vi "Set Home State.vi"(8 "error in (no error)":errorcluster, 9 "Home?":bool, 10 "Motor":i32, 11 "Filter Wheel in":refnum<class "Filter Wheel.lvclass">) -> (0 "error out":errorcluster, 3 "Filter Wheel out":refnum<class "Filter Wheel.lvclass">)   [LabVIEW 2024, in "Filter Wheel.lvclass"]
uses:
  Filter Wheel.lvclass
  Filter Wheel.lvclass/Filter Wheel.ctl
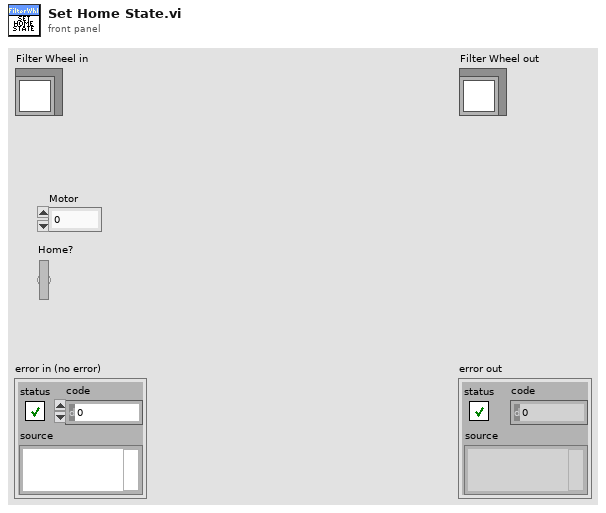
[diagram p1: front panel]
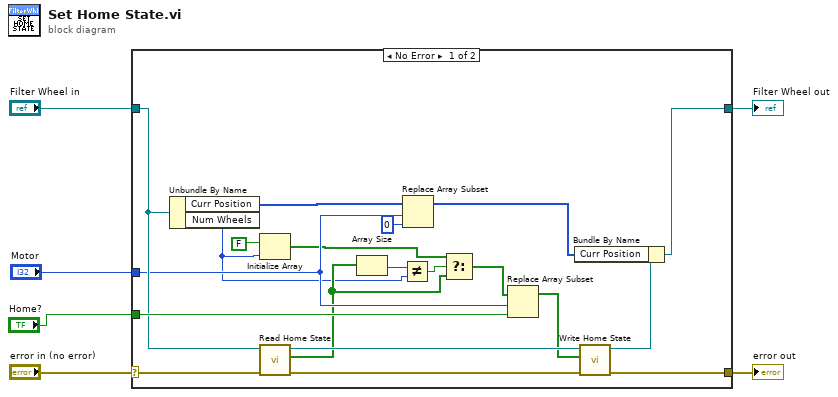
[diagram p0: block diagram]
diagram:
  n1 = case shown="No Error" "error in (no error)" {
    selector: "error in (no error)" -> [w24 w28]
    tunnel: [w22 w28] -> w5
    tunnel: [w19 w27] -> w3
    tunnel: "Filter Wheel in" -> [w18 w27]
    tunnel: "Motor" -> [w16 _]
    tunnel: "Home?" -> [w21 _]
    frame No Error {
      n2 = Unbundle By Name(w18) -> ("Curr Position"=w17:i32[], "Num Wheels"=w7:i32)
      n3 = Initialize Array(FALSE, w7) -> (w8:bool[])
      n4 = call-dynamic "Read Home State.vi"("error in (no error)"=w24, "Filter Wheel in"=w18) -> ("error out"=w23:errorcluster, "Home State"=w11:bool[], "Filter Wheel out"=w26:refnum<class "Filter Wheel.lvclass">)  [unwired: 7 in]
      n5 = Array Size(array=w11) -> (size(s)=w13:i32)
      n6 = Not Equal?(x=w13, y=w7) -> (x != y?=w12:bool)
      n7 = Replace Array Subset(array=w17, new element=0 ("new element/subarray"), index=w16) -> (w14:i32[])
      n8 = Select(t=w8, s=w12, f=w11) -> (s? t:f=w10:bool[])
      n9 = Replace Array Subset(array=w10, new element=w21, index=w16) -> (w25:bool[])
      n10 = call-dynamic "Write Home State.vi"("error in (no error)"=w23, "Home State"=w25, "Filter Wheel in"=w26) -> ("error out"=w22:errorcluster, "Filter Wheel out"=w20:refnum<class "Filter Wheel.lvclass">)  [unwired: 7 in]
      n11 = Bundle By Name(cluster=w20, "Curr Position"=w14) -> (w19:refnum<class "Filter Wheel.lvclass">)
    }
    frame Error {
    }
  }
  "error out" <- w5
  "Filter Wheel out" <- w3
